vi "Review Recipe for Overlap.vi"(6 "Waypoints":cluster{"x":dbl, "y":dbl, "th":dbl}[](array[cluster]), 8 "Blends":T1[](array[typedef]), 11 "Min R":dbl[](array[numeric])) -> (0 "Blends out":T1[](array[typedef]), 2 "Linear Info":T2(array[cluster]), 3 "Length (f)":dbl, 4 "Waypoints out":cluster{"x":dbl, "y":dbl, "th":dbl}[](array[cluster]))   [LabVIEW 2019]
uses:
  BlendType.ctl
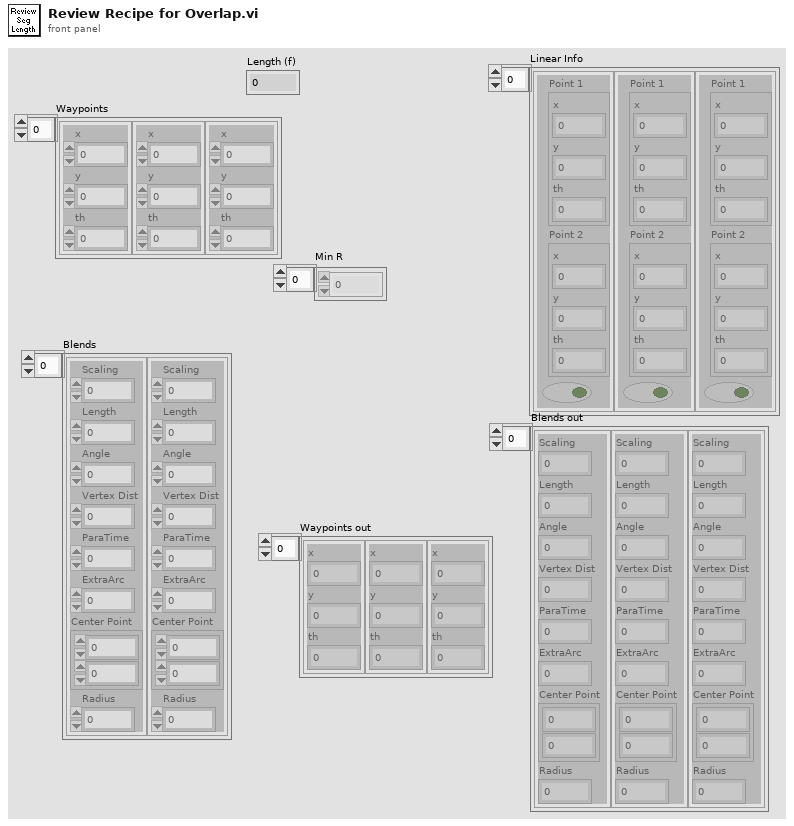
[diagram p1: front panel]
types:
  T1 = typedef "BlendType.ctl" = cluster{"Scaling":dbl, "Length":dbl, "Angle":dbl, "Vertex Dist":dbl, "ParaTime":dbl, "ExtraArc":dbl, "Center Point":cluster{dbl, dbl}, "Radius":dbl}
  T2 = cluster{"Point 1":cluster{"x":dbl, "y":dbl, "th":dbl}, "Point 2":cluster{"x":dbl, "y":dbl, "th":dbl}, bool}[]
  T3 = cluster{"Point Out":cluster{"x":dbl, "y":dbl, "th":dbl}, "Point Out":cluster{"x":dbl, "y":dbl, "th":dbl}, bool}
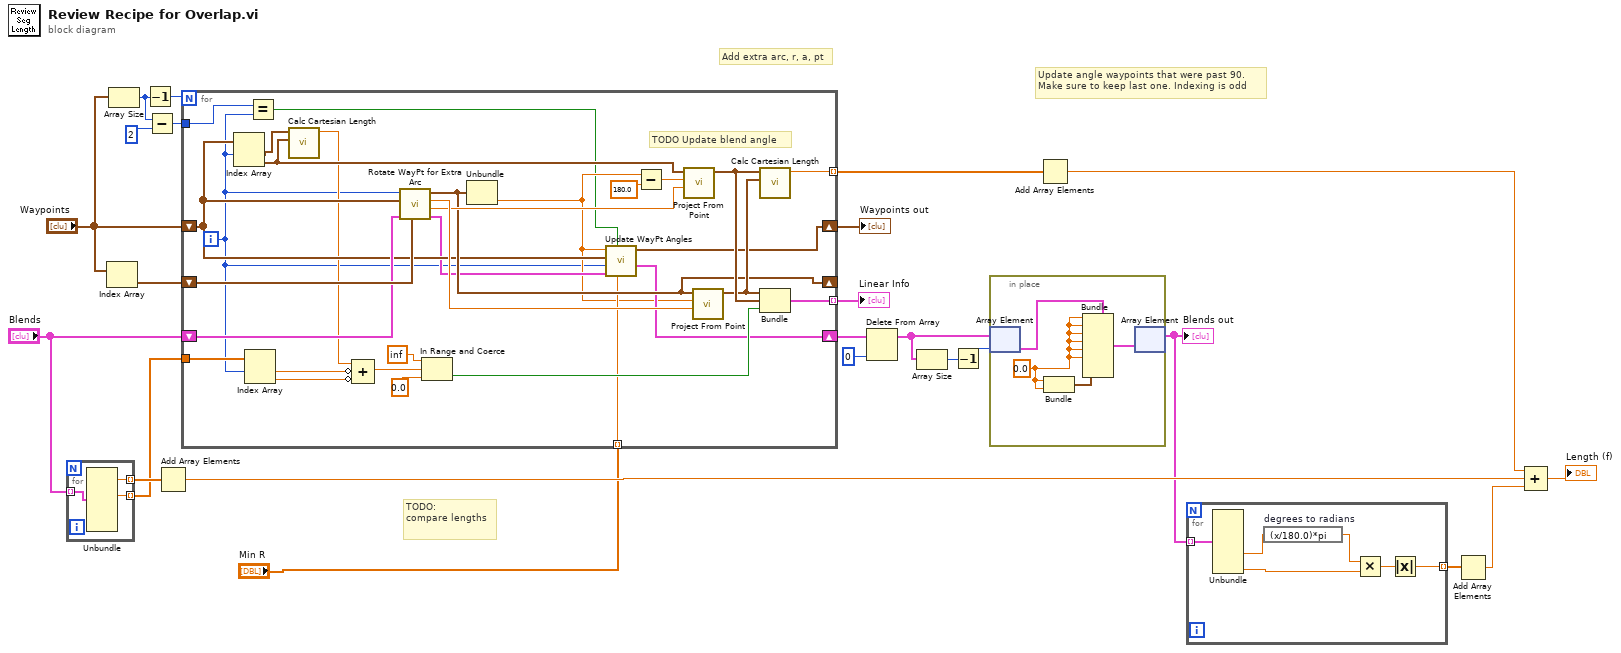
[diagram p0: block diagram]
diagram:
  # "TODO:\ncompare lengths"
  # "Update angle waypoints that were past 90.\nMake sure to keep last one. Indexing is odd"
  # "Add extra arc, r, a, pt"
  n1 = for {
    tunnel: "Blends" -> [w27] mode=indexing
    tunnel: [w26] -> w15 mode=indexing
    tunnel: [w25] -> w14 mode=indexing
    n2 = Unbundle(w27) -> ("Length"=w26:dbl, "Vertex Dist"=w25:dbl)  [unwired: 6 out]
  }
  n3 = Index Array(array="Waypoints") -> (element=w20:cluster{"x":dbl, "y":dbl, "th":dbl})  [unwired: 1 in]
  n4 = Array Size(array="Waypoints") -> (size(s)=w7:i32)
  n5 = Decrement(x=w7) -> (x-1=w17:i32)
  n6 = Subtract(x=w7, y=2 ("index")) -> (x-y=w5:i32)
  n7 = Add Array Elements(numeric array=w15) -> (sum=w13:dbl)
  n8 = for {
    N: w17 -> [_]
    tunnel: [w57] -> w23 mode=indexing
    tunnel: [w52] -> w24 mode=indexing
    shift-right: [w47] -> _
    shift-left: w20 -> [w51]
    shift-right: [w33] -> w22
    shift-left: "Blends" -> [w50]
    shift-right: [w45] -> w19
    shift-left: "Waypoints" -> [w46]
    tunnel: w14 -> [w44]
    tunnel: "Min R" -> [w32] mode=indexing
    tunnel: w5 -> [w30]
    i -> [w29]
    # "TODO Update blend angle"
    n9 = Index Array(array=w46, index #1=w29) -> (element #1=w43:cluster{"x":dbl, "y":dbl, "th":dbl}, element #2=w42:cluster{"x":dbl, "y":dbl, "th":dbl})  [unwired: 1 in]
    n10 = Index Array(array=w44, index #1=w29) -> (element #1=w39:dbl, element #2=w40:dbl)  [unwired: 1 in]
    n11 = Equal?(x=w30, y=w29) -> (x = y?=w28:bool)
    n12 = call "Calc Cartesian Length.vi"("Point 2"=w42, "Point 1"=w43) -> ("Length (f)"=w41:dbl)  [unwired: 8 in, 1 out]
    n13 = Compound Arithmetic op=ADD(w41, invert w39, invert w40) -> (w38:dbl)
    n14 = call "Rotate WayPt for Extra Arc.vi"("Pt 0"=w51, "Blends In"=w50, "Pts"=w46, "index"=w29) -> ("Blends Out"=w34:T1[], "Pt2 vertex dist"=w48:dbl, "Pt0 vertex dist"=w49:dbl, "Pt Out"=w47:cluster{"x":dbl, "y":dbl, "th":dbl})  [unwired: 4 in]
    n15 = In Range and Coerce(upper limit=inf, x=w38, lower limit=0.0 ("upper limit")) -> (In Range?=w35:bool)  [unwired: 1 out]
    n16 = Unbundle(w47) -> ("th"=w31:dbl)  [unwired: 2 out]
    n17 = call "Update WayPt Angles.vi"("Min R"=w32, "Propagate"=w28, "Blends In"=w34, "Index"=w29, "Waypoints in"=w46, "th"=w31) -> ("Blends Out"=w33:T1[], "Waypoints out"=w45:cluster{"x":dbl, "y":dbl, "th":dbl}[])  [unwired: 4 in]
    n18 = Subtract(x=w31, y=180.0) -> (x-y=w56:dbl)
    n19 = call "Project From Point.vi"("distance"=w48, "th"=w56, "Point In"=w42) -> ("Point Out"=w54:cluster{"x":dbl, "y":dbl, "th":dbl})  [unwired: 8 in]
    n20 = call "Project From Point.vi"("distance"=w49, "th"=w31, "Point In"=w47) -> ("Point Out"=w53:cluster{"x":dbl, "y":dbl, "th":dbl})  [unwired: 8 in]
    n21 = call "Calc Cartesian Length.vi"("Point 2"=w53, "Point 1"=w54) -> ("Length (f)"=w52:dbl)  [unwired: 8 in, 1 out]
    n22 = Bundle("Point Out"=w53, "Point Out"=w54, w35) -> (w57:T3)  [unwired: 1 in]
  }
  "Linear Info" <- w23
  "Waypoints out" <- w19
  n23 = Delete From Array(array=w22, index=0) -> (array with subset deleted=w4:T1[])  [unwired: 1 in, 1 out]
  n24 = Array Size(array=w4) -> (size(s)=w9:i32)
  n25 = Decrement(x=w9) -> (x-1=w8:i32)
  n26 = in-place {
    w59 = 0.0 ("ExtraArc")
    n27 = in-place-array #1(w4, w8) -> (w61:T1)
    n28 = Bundle("ExtraArc"=w59, "ExtraArc"=w59) -> (w58:cluster{"ExtraArc":dbl, "ExtraArc":dbl})  [unwired: 1 in]
    n29 = Bundle(cluster=w61, "Scaling"=w59, "Length"=w59, "Angle"=w59, "Vertex Dist"=w59, "ParaTime"=w59, "ExtraArc"=w59, "Center Point"=w58) -> (w60:T1)  [unwired: 1 in]
    n30 = in-place-array #1(w60) -> (w1:T1[])  [unwired: 1 out]
  }
  "Blends out" <- w1
  n31 = Add Array Elements(numeric array=w24) -> (sum=w12:dbl)
  n32 = for {
    tunnel: w1 -> [w67] mode=indexing
    tunnel: [w62] -> w3 mode=indexing
    n33 = Unbundle(w67) -> ("ExtraArc"=w65:dbl, "Radius"=w66:dbl)  [unwired: 6 out]
    n34 = expression code="(x/180.0)*pi" "degrees to radians"(w65) -> (w64:dbl)
    n35 = Multiply(x=w64, y=w66) -> (x*y=w63:dbl)
    n36 = Absolute Value(x=w63) -> (abs(x)=w62:dbl)
  }
  n37 = Add Array Elements(numeric array=w3) -> (sum=w2:dbl)
  n38 = Compound Arithmetic op=ADD(w12, w13, w2) -> (→"Length (f)":dbl)
